vi "Centauro Verify Display.vi"(0 "GEA2 Reference In":refnum<k24>, 5 "Standalone?":bool, 7 "Expected LED Status":T3, 9 "Care":T1, 11 "Error In":errorcluster) -> (4 "GEA2 Reference Out":refnum<k24>, 6 "Pass/Fail?":bool=TRUE, 8 "Report Text":string, 10 "Binary Number Out":u32, 15 "Error Out":errorcluster)   [LabVIEW 2016]
uses:
  Q:/Common/DLLs/GEA3/GeaCommunication.dll
  Common/DLLs/GEA3/GeaCommunication.dll
  type defs/LED Status OOB.ctl
  Common/LabVIEW GEA2 Toolkit/LabVIEW_GEA2_Toolkit.lvlibp/type defs/Source_Destination.ctl
  Common/LabVIEW GEA2 Toolkit/LabVIEW_GEA2_Toolkit.lvlibp/type defs/ERD Read Data In.ctl
  Common/LabVIEW GEA2 Toolkit/LabVIEW_GEA2_Toolkit.lvlibp/type defs/Data Type.ctl
  Common/LabVIEW GEA2 Toolkit/LabVIEW_GEA2_Toolkit.lvlibp
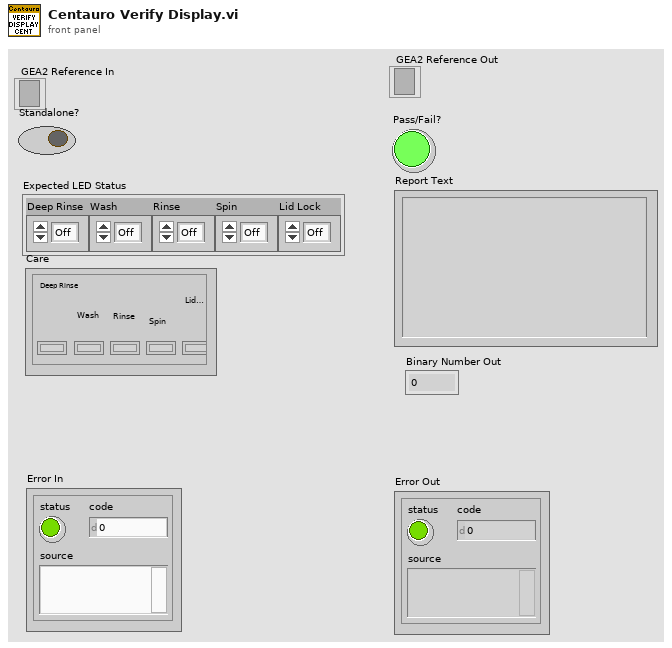
[diagram p1: front panel]
types:
  T1 = cluster{"Deep Rinse":bool, "Wash":bool, "Rinse":bool, "Spin":bool, "Lid Lock":bool}
  T2 = typedef "LED Status OOB.ctl" = enum32{"Off", "On", "Blink"}
  T3 = cluster{"Deep Rinse":T2, "Wash":T2, "Rinse":T2, "Spin":T2, "Lid Lock":T2}
  T4 = typedef "LabVIEW_GEA2_Toolkit.lvlibp/ERD Read Data In.ctl" = cluster{"ERD Number":u16, "Data Type":T5}
  T5 = typedef "LabVIEW_GEA2_Toolkit.lvlibp/Data Type.ctl" = enum16{"string", "boolean", "uint8_t", "uint16_t", "uint32_t", "uint64_t", "int8_t", "int16_t", "int32_t", "int64_t"}
  T6 = typedef "LabVIEW_GEA2_Toolkit.lvlibp/Source_Destination.ctl" = cluster{"Source":u8, "Destination":u8}
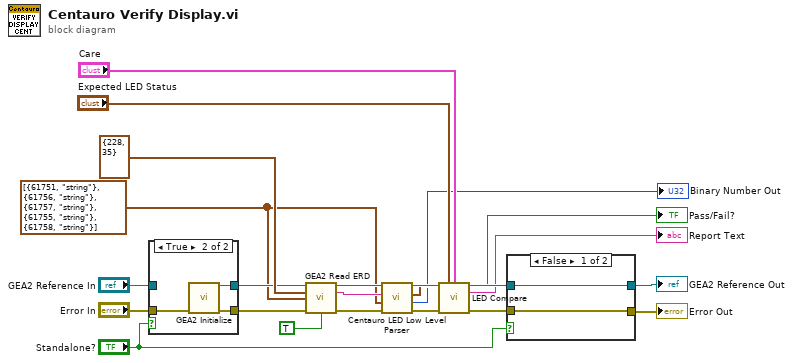
[diagram p0: block diagram]
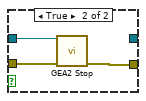
[diagram p2: hidden frame]
diagram:
  w8 = T4[] [{"ERD Number"=61751, "Data Type"=enum."string"}, {"ERD Number"=61756, "Data Type"=enum."string"}, {"ERD Number"=61757, "Data Type"=enum."string"}, {"ERD Number"=61755, "Data Type"=enum."string"}, {"ERD Number"=61758, "Data Type"=enum."string"}] ("Read ERD List")
  n1 = case shown="True" "Standalone?" {
    tunnel: [w22 w26] -> w19
    tunnel: "Error In" -> [w22 w25]
    tunnel: [w23 w24] -> w17
    tunnel: "GEA2 Reference In" -> [w23 _]
    frame False {
    }
    frame True {
      n2 = call "GEA2 Initialize.vi"("error in"=w25) -> ("GEA2 Reference Out"=w24:refnum<k24>, "error out"=w26:errorcluster)  [unwired: 12 in, 1 out]
    }
  }
  n3 = call "GEA2 Read ERD.vi"("GEA2 Reference In"=w17, "GEA Inputs"=T6 {"Source"=228, "Destination"=35}, "Read ERD List"=w8, "Error In"=w19, "Verify ERD Response?"=TRUE) -> ("GEA2 Reference Out"=w12:refnum<k24>, "Raw Data Out"=w9:string, "Error Out"=w4:errorcluster)  [unwired: 7 in, 1 out]
  n4 = call "Centauro LED Low Level Parser.vi"("error in (no error)"=w4, "Read ERD List"=w8, "Raw Data In"=w9) -> ("error out"=w11:errorcluster, "Binary Number"=→"Binary Number Out":u32, "LED Status"=w10:T3)  [unwired: 6 in]
  n5 = call "LED Compare.vi"("Actul LED Status"=w10, "Expected LED Status"="Expected LED Status", "Care"="Care", "Error In"=w11) -> ("Pass/Fail?"=→"Pass/Fail?":bool, "Report Text"=→"Report Text":string, "Error Out"=w5:errorcluster)  [unwired: 9 in]
  n6 = case shown="False" "Standalone?" {
    tunnel: [w27 w31] -> w15
    tunnel: [w28 _] -> w13
    tunnel: w12 -> [w28 w30]
    tunnel: w5 -> [w27 w29]
    frame False {
    }
    frame True {
      n7 = call "GEA2 Stop.vi"("GEA2 Reference In"=w30, "Error In"=w29) -> ("Error Out"=w31:errorcluster)  [unwired: 13 in]
    }
  }
  "GEA2 Reference Out" <- w13
  "Error Out" <- w15
